vi "Read Parent Attributes.vi"(11 "Spawn in":refnum<class "Spawn.lvclass">) -> (2 "Parent Attributes":refnum<class "Attributes.lvclass">)   [LabVIEW 2025, in "jettl.lvlib" / "Spawn.lvlib" / "Spawn.lvclass"]
uses:
  Spawn.lvclass
  Attributes/Attributes/Attributes.lvclass
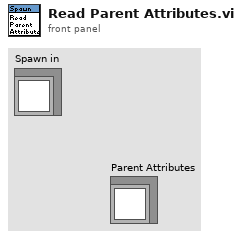
[diagram p1: front panel]
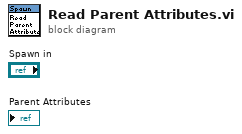
[diagram p0: block diagram]
diagram:
